vi "Impureza sript.vi"(0 "Image In":T1, 1 "Image Dst":T1, 7 "error in":errorcluster) -> (20 "Image Out":T1, 21 "Straight Edge (Find Straight Edge 1)":T4 {"Point2 (Real-World)"."Y" format="%.2f"; "Point2 (Real-World)"."X" format="%.2f"; "Point1 (Real-World)"."Y" format="%.2f"; "Point1 (Real-World)"."X" format="%.2f"; "Point2 (Pixels)"."Y" format="%.2f"; "Point2 (Pixels)"."X" format="%.2f"; "Point1 (Pixels)"."Y" format="%.2f"; "Point1 (Pixels)"."X" format="%.2f"}, 22 "Straight Edge (Copy of Find Straight Edge 1)":T4 {"Point2 (Real-World)"."Y" format="%.2f"; "Point2 (Real-World)"."X" format="%.2f"; "Point1 (Real-World)"."Y" format="%.2f"; "Point1 (Real-World)"."X" format="%.2f"; "Point2 (Pixels)"."Y" format="%.2f"; "Point2 (Pixels)"."X" format="%.2f"; "Point1 (Pixels)"."Y" format="%.2f"; "Point1 (Pixels)"."X" format="%.2f"}, 27 "error out":errorcluster)   [LabVIEW 2020]
doc: "Creates, edits, and runs vision algorithms using NI Vision Assistant.\n\nWhen you place this Express VI on the block diagram, NI Vision Assistant launches. Create an algorithm using the Vision Assistant processing functions. After you create an algorithm, you can select the controls and indicators that you want to be able to programmatically set in LabVIEW. Double-click the Vision Assistant Express VI to edit the algorithm."
uses:
  <vilib>/vision/Image Controls.llb/IMAQ Image.ctl
  <vilib>/vision/Measure.llb/Edge Options.ctl
  <vilib>/vision/Measure.llb/Edge Polarity.ctl
  <vilib>/vision/Measure.llb/Straight Edge Options.ctl
  <vilib>/vision/Measure.llb/Straight Edge Process.ctl
  <vilib>/vision/NI_Vision_Development_Module.lvlib
panel:
  out "Image Out 3":T1(plugin-control)
  out "Straight Edges 2":T2(array[cluster]) {"Point2 (Real-World)"."Y" format="%.2f"; "Point2 (Real-World)"."X" format="%.2f"; "Point1 (Real-World)"."Y" format="%.2f"; "Point1 (Real-World)"."X" format="%.2f"; "Point2 (Pixels)"."Y" format="%.2f"; "Point2 (Pixels)"."X" format="%.2f"; "Point1 (Pixels)"."Y" format="%.2f"; "Point1 (Pixels)"."X" format="%.2f"}
  out "Straight Edges":T2(array[cluster]) {"Point2 (Real-World)"."Y" format="%.2f"; "Point2 (Real-World)"."X" format="%.2f"; "Point1 (Real-World)"."Y" format="%.2f"; "Point1 (Real-World)"."X" format="%.2f"; "Point2 (Pixels)"."Y" format="%.2f"; "Point2 (Pixels)"."X" format="%.2f"; "Point1 (Pixels)"."Y" format="%.2f"; "Point1 (Pixels)"."X" format="%.2f"}
  out "Coordinate System (duplicate)":T3 {"Measurement System"."Axis Reference" items=["Direct", "Indirect"]; "Measurement System"."Angle (deg)" format="%.2f"; "Measurement System"."Origin"."Y" format="%.2f"; "Measurement System"."Origin"."X" format="%.2f"; "Reference System"."Axis Reference" items=["Direct", "Indirect"]; "Reference System"."Angle (deg)" format="%.2f"; "Reference System"."Origin"."Y" format="%.2f"; "Reference System"."Origin"."X" format="%.2f"}
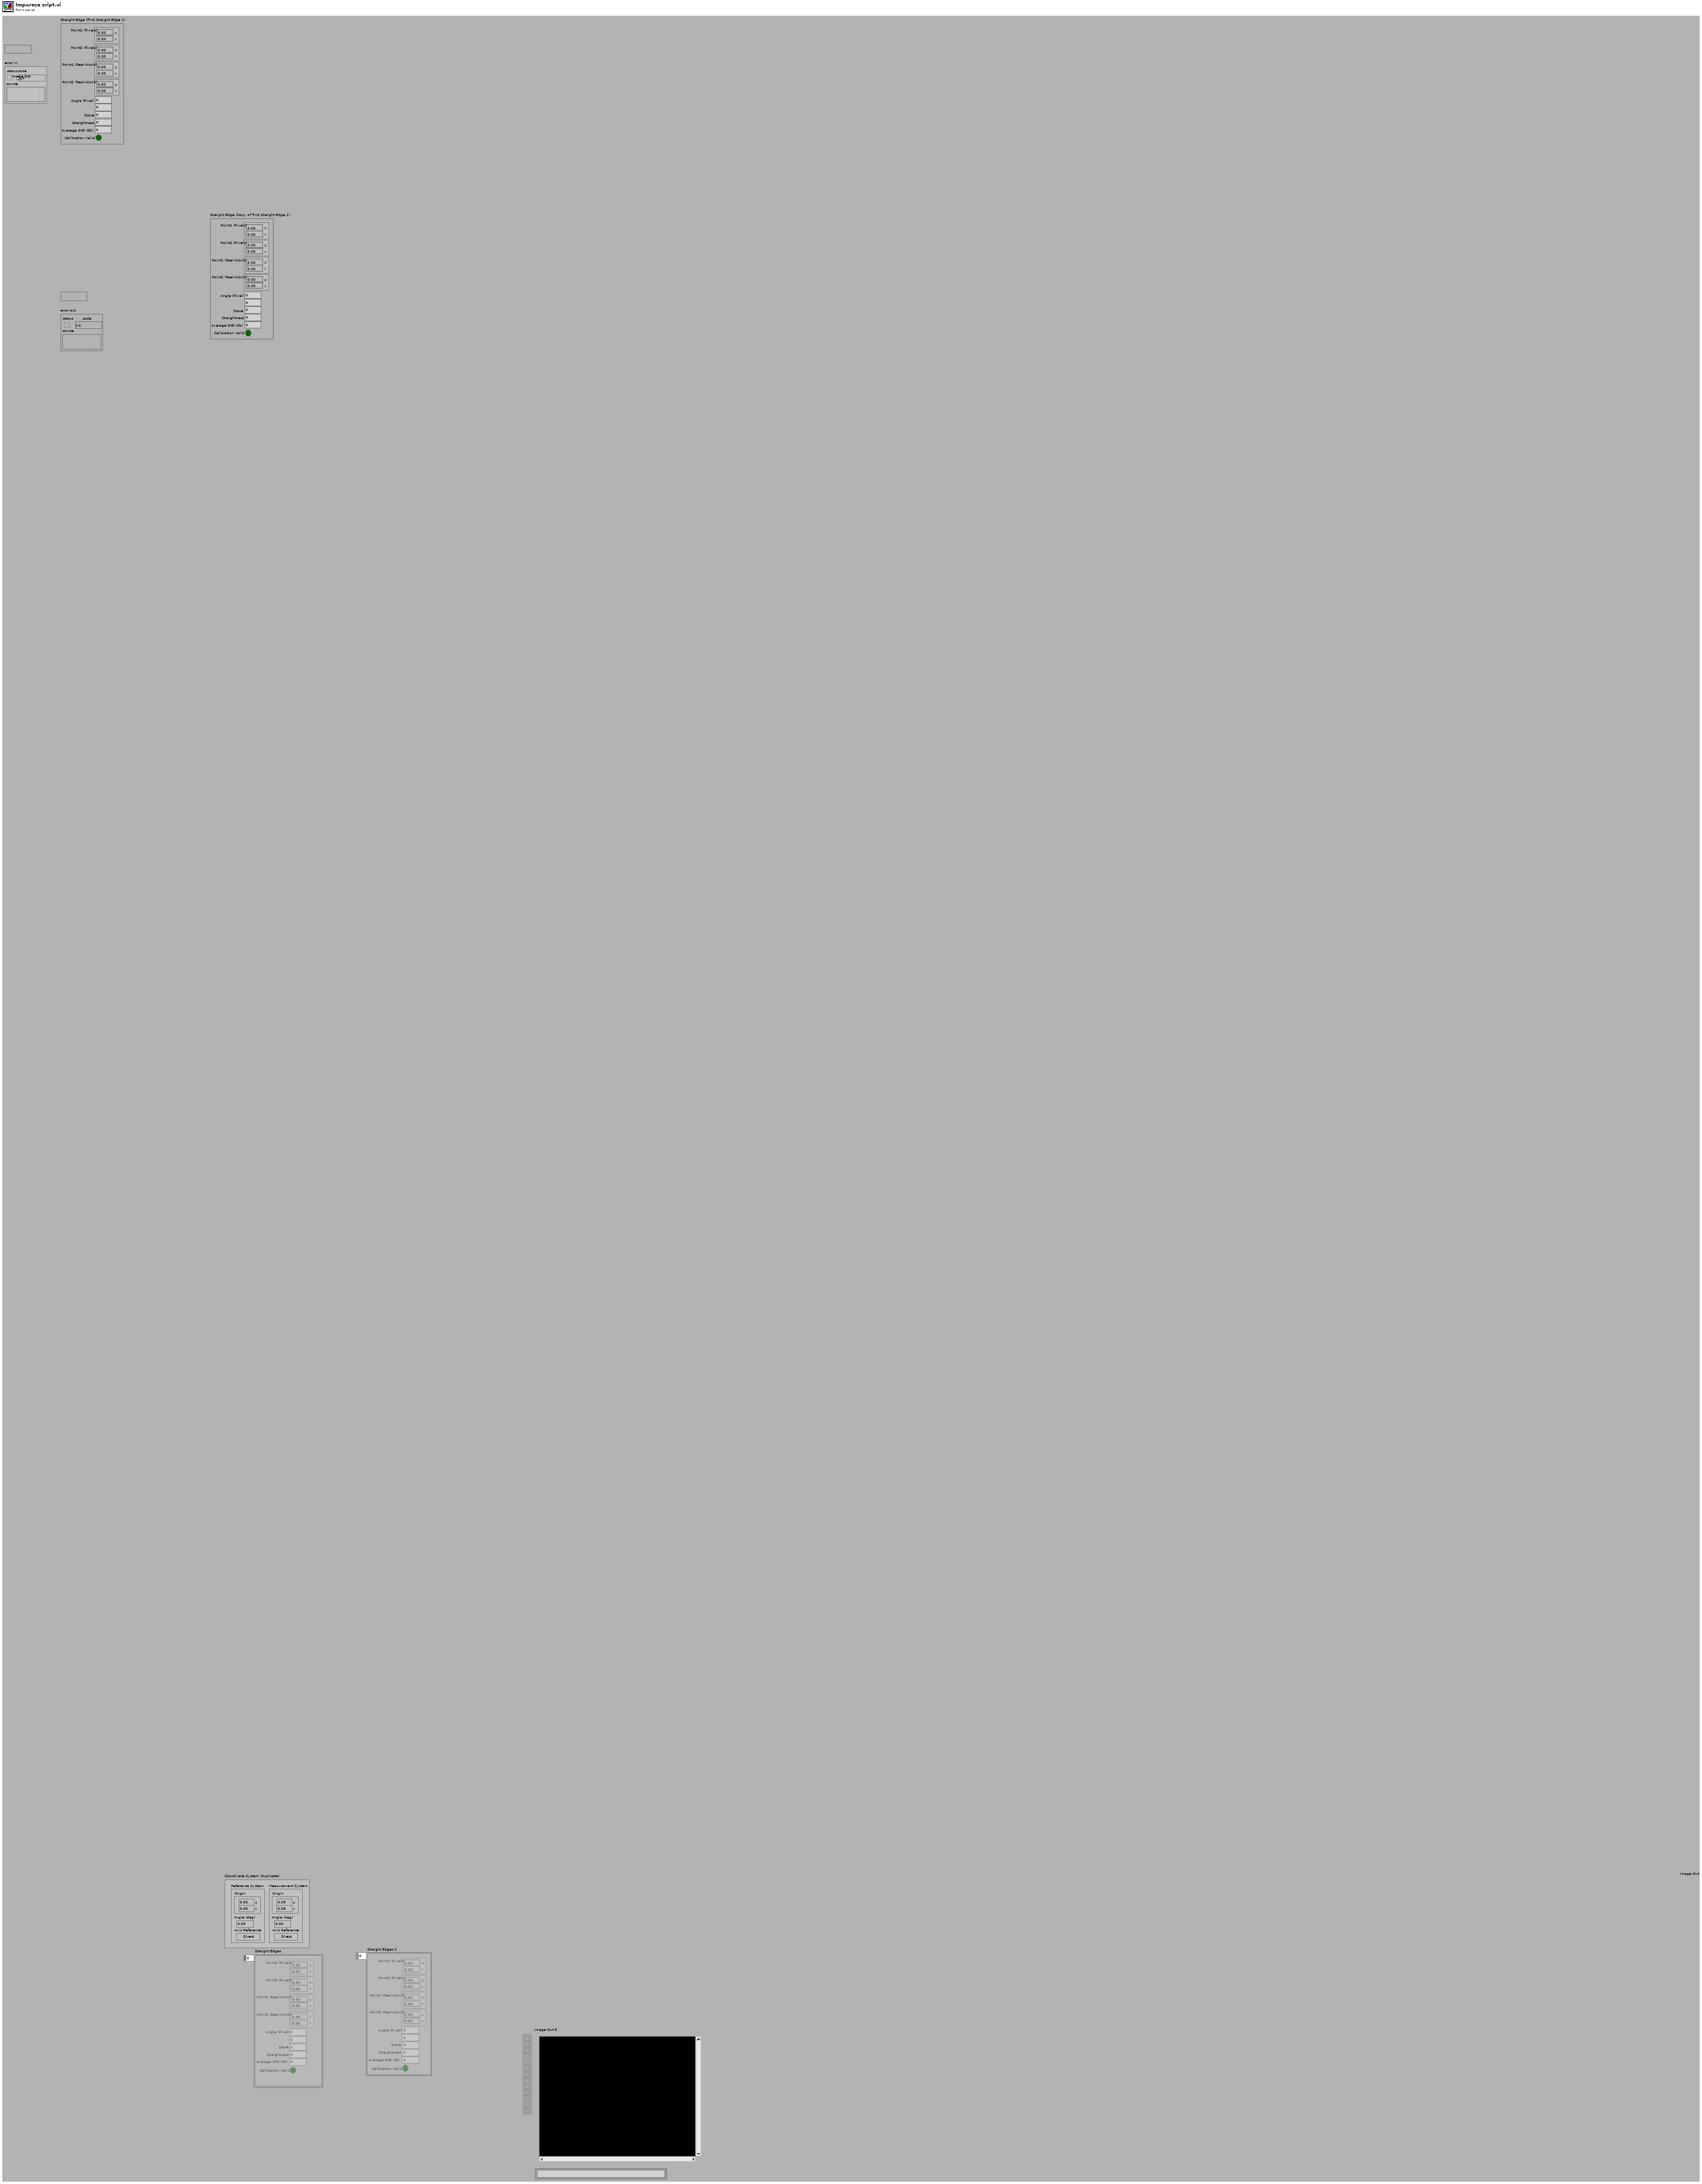
[diagram p1: front panel]
types:
  T1 = typedef "IMAQ Image.ctl" = refnum<image>
  T2 = cluster{"Point1 (Pixels)":cluster{"X":sgl, "Y":sgl}, "Point2 (Pixels)":cluster{"X":sgl, "Y":sgl}, "Point1 (Real-World)":cluster{"X":sgl, "Y":sgl}, "Point2 (Real-World)":cluster{"X":sgl, "Y":sgl}, "Angle (Pixel)":dbl, "Angle (Real-World)":dbl, "Score":dbl, "Straightness":dbl, "Average SNR (db)":dbl, "Calibration Valid":bool}[]
  T3 = typedef "IMAQ Coordinate System" = cluster{"Reference System":cluster{"Origin":cluster{"X":sgl, "Y":sgl}, "Angle (deg)":sgl, "Axis Reference":u32}, "Measurement System":cluster{"Origin":cluster{"X":sgl, "Y":sgl}, "Angle (deg)":sgl, "Axis Reference":u32}}
  T4 = cluster{"Point1 (Pixels)":cluster{"X":sgl, "Y":sgl}, "Point2 (Pixels)":cluster{"X":sgl, "Y":sgl}, "Point1 (Real-World)":cluster{"X":sgl, "Y":sgl}, "Point2 (Real-World)":cluster{"X":sgl, "Y":sgl}, "Angle (Pixel)":dbl, "Angle (Real-World)":dbl, "Score":dbl, "Straightness":dbl, "Average SNR (db)":dbl, "Calibration Valid":bool}
  T5 = typedef "Edge Options.ctl" = cluster{"Edge Polarity":T6, "Kernel Size":u32, "Width":u32, "Minimum Edge Strength":sgl, "Interpolation Type":enum32{"Zero Order", "Bilinear", "Quadratic", "Cubic", "Bilinear Fixed"}, "Data Processing Method":enum32{"Average", "Median"}}
  T6 = typedef "Edge Polarity.ctl" = u32
  T7 = cluster{"Search Direction":u32, "Edge Options":T5, "Show Search Area":bool, "Show Search Lines":bool, "Show Edges Found":bool, "Show Result":bool, "Search Area Color":u32, "Search Lines Color":u32, "Edge Locations Color":u32, "Result Color":u32, "Overlay Group Name":string}
  T8 = typedef "Straight Edge Options.ctl" = cluster{"Number of Lines":i32, "Type":T9, "Min. Score":dbl, "Max. Score":dbl, "Orientation":dbl, "Angle Range":dbl, "Angle Tolerance":dbl, "Step Size":u32, "Min. SNR (db)":dbl, "Min. Points (%)":dbl, "Hough Iterations":i32}
  T9 = typedef "Straight Edge Process.ctl" = enum32{"First Edge Rake", "Best Edge Rake", "Hough Edge Rake", "First Edge Projection", "Best Edge Projection"}
  T10 = cluster{"Global Rectangle":i32[], "Contours":cluster{"ID":enum32{"External", "Internal"}, "Type":u32, "Coordinates":i32[]}[]}
  T11 = typedef "Image Type" = u32
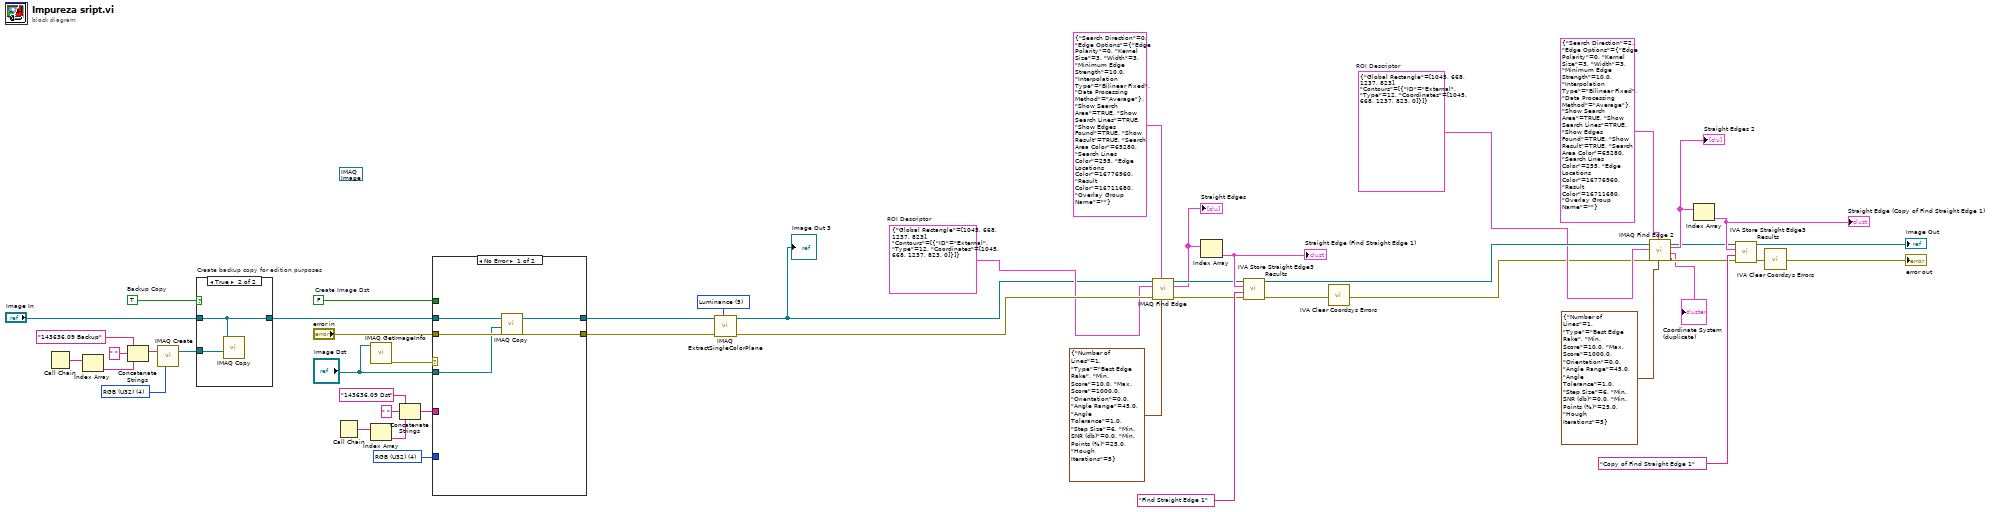
[diagram p0: block diagram]
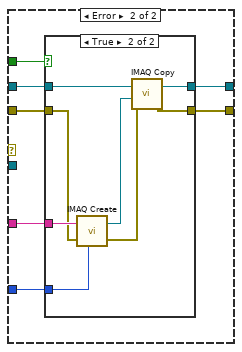
[diagram p2: hidden frame]
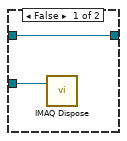
[diagram p4: hidden frame]
diagram:
  (unwired) T1 refnum ("Image Out 3")
  w8 = T10 {"Global Rectangle"=[1045, 668, 1237, 823], "Contours"=[{"ID"=enum."External", "Type"=12, "Coordinates"=[1045, 668, 1237, 823, 0]}]}  # ROI Descriptor
  w24 = T10 {"Global Rectangle"=[1045, 668, 1237, 823], "Contours"=[{"ID"=enum."External", "Type"=12, "Coordinates"=[1045, 668, 1237, 823, 0]}]}  # ROI Descriptor
  w27 = 5 items=["Red", "Green", "Blue", "Hue", "Saturation", "Luminance", "Value", "Intensity"] ("Color Plane")
  w28 = T11 4 items=["Grayscale (U8)", "Grayscale (I16)", "Grayscale (SGL)", "Complex (CSG)", "RGB (U32)", "HSL (U32)", "RGB (U64)", "Grayscale (U16)"] ("Image Dst Type")
  w29 = T11 4 items=["Grayscale (U8)", "Grayscale (I16)", "Grayscale (SGL)", "Complex (CSG)", "RGB (U32)", "HSL (U32)", "RGB (U64)", "Grayscale (U16)"] ("Image Type")
  w48 = TRUE  # Backup Copy
  w41 = FALSE  # Create Image Dst
  n1 = Call Chain() -> (call chain=w35:string[])
  n2 = Index Array(array=w35) -> (element=w34:string)  [unwired: 1 in]
  n3 = Concatenate Strings("143636,09 Backup" ("Backup Image Name"), " ", w34) -> (w31:string)
  n4 = call "IMAQ Create"("Image Name"=w31, "Image Type"=w29) -> ("New Image"=w30:T1)  [unwired: 2 in, 2 out]
  n5 = case "Create backup copy for edition purposes" shown="True" w48 {
    tunnel: [w50 w52] -> w44
    tunnel: "Image In" -> [w50 w52]
    tunnel: w30 -> [w49 w51]
    frame False {
      n6 = call "IMAQ Dispose"("Image"=w49) -> ()  [unwired: 2 in, 4 out]
    }
    frame True {
      n7 = call "IMAQ Copy"("Image Dst"=w51, "Image Src"=w52) -> ()  [unwired: 1 in, 5 out]
    }
  }
  n8 = Call Chain() -> (call chain=w40:string[])
  n9 = call "IMAQ GetImageInfo"("Image"="Image Dst") -> ("error out"=w46:errorcluster)  [unwired: 1 in, 9 out]
  n10 = Index Array(array=w40) -> (element=w38:string)  [unwired: 1 in]
  n11 = Concatenate Strings("143636,09 Dst" ("Image Dst Name"), " ", w38) -> (w36:string)
  n12 = case shown="No Error" w46 {
    tunnel: [w57 w61] -> w26
    tunnel: [w56 w60] -> w42
    tunnel: w44 -> [w55 w62]
    tunnel: "error in" -> [w54 w58]
    tunnel: "Image Dst" -> [w53 _]
    tunnel: w36 -> [_ w64]
    tunnel: w28 -> [_ w63]
    tunnel: w41 -> [_ w59]
    frame No Error {
      n13 = call "IMAQ Copy"("error in (no error)"=w54, "Image Dst"=w53, "Image Src"=w55) -> ("error out"=w56:errorcluster, "Image Dst Out"=w57:T1)  [unwired: 3 out]
    }
    frame Error {
      n14 = case shown="True" w59 {
        tunnel: w64 -> [_ w74]
        tunnel: w63 -> [_ w73]
        tunnel: w62 -> [w66 w71]
        tunnel: [w66 w70] -> w61
        tunnel: [w65 w69] -> w60
        tunnel: w58 -> [w65 w67]
        frame False {
        }
        frame True {
          n15 = call "IMAQ Create"("Image Name"=w74, "Image Type"=w73, "error in (no error)"=w67) -> ("New Image"=w72:T1, "error out"=w68:errorcluster)  [unwired: 1 in, 1 out]
          n16 = call "IMAQ Copy"("error in (no error)"=w68, "Image Dst"=w72, "Image Src"=w71) -> ("error out"=w69:errorcluster, "Image Dst Out"=w70:T1)  [unwired: 3 out]
        }
      }
    }
  }
  n17 = call "IMAQ ExtractSingleColorPlane"("Color Plane"=w27, "error in (no error)"=w42, "Image Src"=w26) -> ("error out"=w25:errorcluster, "Image Dst Out"=w1:T1)  [unwired: 1 in, 6 out]
  "Image Out 3" <- w1
  n18 = call "IMAQ Find Edge"("Line Fit Options"=T8 {"Number of Lines"=1, "Type"=enum."Best Edge Rake", "Min. Score"=10.0, "Max. Score"=1000.0, "Orientation"=0.0, "Angle Range"=45.0, "Angle Tolerance"=1.0, "Step Size"=6, "Min. SNR (db)"=0.0, "Min. Points (%)"=25.0, "Hough Iterations"=5} ("Fit Options"), "Options"=T7 {"Search Direction"=0, "Edge Options"={"Edge Polarity"=0, "Kernel Size"=3, "Width"=3, "Minimum Edge Strength"=10.0, "Interpolation Type"=enum."Bilinear Fixed", "Data Processing Method"=enum."Average"}, "Show Search Area"=TRUE, "Show Search Lines"=TRUE, "Show Edges Found"=TRUE, "Show Result"=TRUE, "Search Area Color"=65280, "Search Lines Color"=255, "Edge Locations Color"=16776960, "Result Color"=16711680, "Overlay Group Name"=""}, "error in (no error)"=w25, "ROI Descriptor"=w24, "Image"=w1) -> ("error out"=w18:errorcluster, "Straight Edges"=w17:T2, "Image Out"=w19:T1)  [unwired: 1 in, 3 out]
  "Straight Edges" <- w17
  n19 = Index Array(array=w17) -> (element=w20:T4)  [unwired: 1 in]
  "Straight Edge (Find Straight Edge 1)" <- w20
  n20 = call <vilib>:"IVA Store Straight Edge3 Results.vi"("error in (no error)"=w18, "Step Name"="Find Straight Edge 1", "Straight Edge"=w20, "Image in"=w19) -> ("error out"=w16:errorcluster, "Image dup"=w9:T1)  [unwired: 1 in, 5 out]
  n21 = call <vilib>:"IVA Clear Coordsys Errors.vi"("error in (no error)"=w16) -> ("error out"=w7:errorcluster)  [unwired: 10 in]
  n22 = call "IMAQ Find Edge 2"("Line Fit Options"=T8 {"Number of Lines"=1, "Type"=enum."Best Edge Rake", "Min. Score"=10.0, "Max. Score"=1000.0, "Orientation"=0.0, "Angle Range"=45.0, "Angle Tolerance"=1.0, "Step Size"=6, "Min. SNR (db)"=0.0, "Min. Points (%)"=25.0, "Hough Iterations"=5} ("Fit Options"), "Options"=T7 {"Search Direction"=2, "Edge Options"={"Edge Polarity"=0, "Kernel Size"=3, "Width"=3, "Minimum Edge Strength"=10.0, "Interpolation Type"=enum."Bilinear Fixed", "Data Processing Method"=enum."Average"}, "Show Search Area"=TRUE, "Show Search Lines"=TRUE, "Show Edges Found"=TRUE, "Show Result"=TRUE, "Search Area Color"=65280, "Search Lines Color"=255, "Edge Locations Color"=16776960, "Result Color"=16711680, "Overlay Group Name"=""}, "error in (no error)"=w7, "ROI Descriptor"=w8, "Image"=w9) -> ("error out"=w5:errorcluster, "Coordinate System (duplicate)"=→"Coordinate System (duplicate)":T3, "Straight Edges"=w3:T2, "Image Out"=w2:T1)  [unwired: 3 in]
  "Straight Edges 2" <- w3
  n23 = Index Array(array=w3) -> (element=w14:T4)  [unwired: 1 in]
  "Straight Edge (Copy of Find Straight Edge 1)" <- w14
  n24 = call <vilib>:"IVA Store Straight Edge3 Results.vi"("error in (no error)"=w5, "Step Name"="Copy of Find Straight Edge 1", "Straight Edge"=w14, "Image in"=w2) -> ("error out"=w13:errorcluster, "Image dup"=→"Image Out":T1)  [unwired: 1 in, 5 out]
  n25 = call <vilib>:"IVA Clear Coordsys Errors.vi"("error in (no error)"=w13) -> ("error out"=→"error out":errorcluster)  [unwired: 10 in]
